vi "GetPigeon2UpTime.vi"(9 "timeoutSeconds":dbl, 10 "WaitForUpdate":bool=TRUE, 11 "DeviceReference":T2) -> (3 "Output":T1)   [LabVIEW 2020]
uses:
  DeviceReference.ctl
  <userlib>/CTRE_PhoenixTools/CTRE_PhoenixTools.lvlib
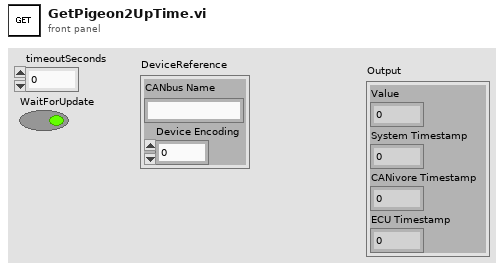
[diagram p1: front panel]
types:
  T1 = cluster{"Value":dbl, "System Timestamp":dbl, "CANivore Timestamp":dbl, "ECU Timestamp":dbl}
  T2 = typedef "DeviceReference.ctl" = cluster{"CANbus Name":string, "Device Encoding":u32}
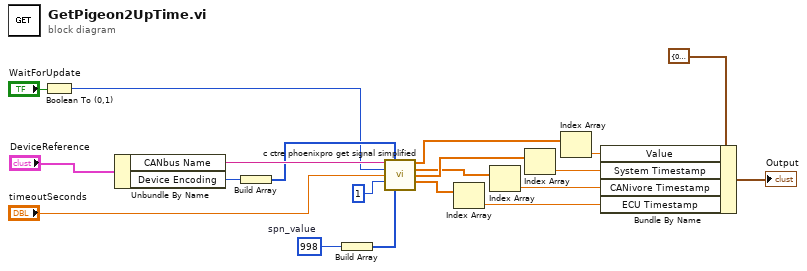
[diagram p0: block diagram]
diagram:
  w11 = u32 998  # spn_value
  n1 = Boolean To (0,1)(Boolean="WaitForUpdate") -> (0, 1=w14:i16)
  n2 = Unbundle By Name("DeviceReference") -> ("CANbus Name"=w19:string, "Device Encoding"=w18:u32)
  n3 = Build Array(w18) -> (w17:u32[])
  n4 = Build Array(w11) -> (w12:u32[])
  n5 = call <userlib>:"c ctre phoenixpro get signal simplified.vi"("network"=w19, "device_hashes"=w17, "bWaitForUpdate"=w14, "timeoutSeconds"="timeoutSeconds", "num_signals"=u32 1, "spns"=w12) -> ("values"=w8:dbl[], "hwTimestampSeconds"=w6:dbl[], "swTimestampSeconds"=w7:dbl[], "ecuTimestampSeconds"=w5:dbl[])  [unwired: 4 in, 2 out]
  n6 = Index Array(array=w5) -> (element=w4:dbl)  [unwired: 1 in]
  n7 = Index Array(array=w6) -> (element=w3:dbl)  [unwired: 1 in]
  n8 = Index Array(array=w7) -> (element=w2:dbl)  [unwired: 1 in]
  n9 = Index Array(array=w8) -> (element=w9:dbl)  [unwired: 1 in]
  n10 = Bundle By Name(cluster=T1 {"Value"=0.0, "System Timestamp"=0.0, "CANivore Timestamp"=0.0, "ECU Timestamp"=0.0} ("Output 2"), "Value"=w9, "System Timestamp"=w2, "CANivore Timestamp"=w3, "ECU Timestamp"=w4) -> (→"Output":T1)
